vi "Create FPGA Data Node.vi"(6 "Path to Analog Node Template":string="IONode\\Analog Input Node x.vi", 7 "Values for Naming":T3={"Bus Number"=1, "Device Number"=1, "Channel Number"=1} {"Channel Number" min=1 step=1; "Device Number" min=1 step=1; "Bus Number" min=1 step=1}, 8 "error in":errorcluster, 10 "Device Information":T1={"Number of Channels"=1, "Device Alias"="", "Icon Text"={"Line 1 text"="Bus", "Line 2 text"="Dev", "Line 3 text"="Ch", "Line 4 text"=""}}, 11 "Path to IO Node":path=path "D:/Documents/Projects/SPIAPI/IOEngineCode") -> (0 "error out":errorcluster, 2 "IO Node Name":string, 3 "Path to new IO Node":path)   [LabVIEW 2014, in "SPI Engine Scripting.lvlib"]
doc: "Creates and saves an IO Node VI. It also modifies the values of its front panel controls based on the \"Values for Naming\" input."
uses:
  SPI Engine Scripting.lvlib
  State Machine/Controls/Values for Naming.ctl
  State Machine/Controls/Device Information.ctl
  <vilib>/LabVIEW Icon API/API_Text.ctl
  Icon Editor/Icon Editor.llb/Icon Colors.ctl
  <vilib>/LabVIEW Icon API/LabVIEW Icon API.lvlib
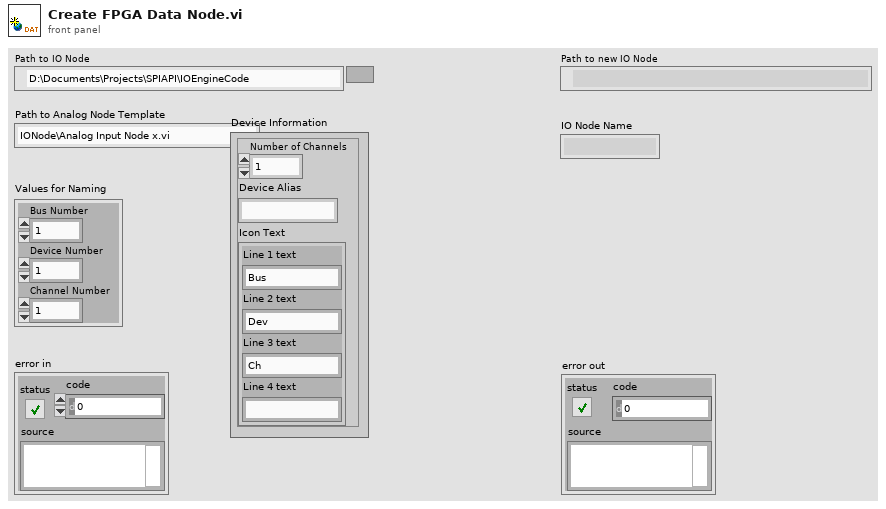
[diagram p1: front panel]
types:
  T1 = typedef "Device Information.ctl" = cluster{"Number of Channels":i32, "Device Alias":string, "Icon Text":T2}
  T2 = typedef "LabVIEW Icon API.lvlib/API_Text.ctl" = cluster{"Line 1 text":string, "Line 2 text":string, "Line 3 text":string, "Line 4 text":string}
  T3 = typedef "SPI Engine Scripting.lvlib/Values for Naming.ctl" = cluster{"Bus Number":i32, "Device Number":i32, "Channel Number":i32}
  T4 = typedef "Icon Colors.ctl" = cluster{"Text Color":u32, "Background Color":u32, "Border Color":u32}
  T5 = enum32{"invalid VI type", "Standard VI", "Control VI", "Global VI", "Polymorphic VI", "Configuration VI", "SubSystem", "Facade VI", "Method VI", "Statechart Diagram VI"}
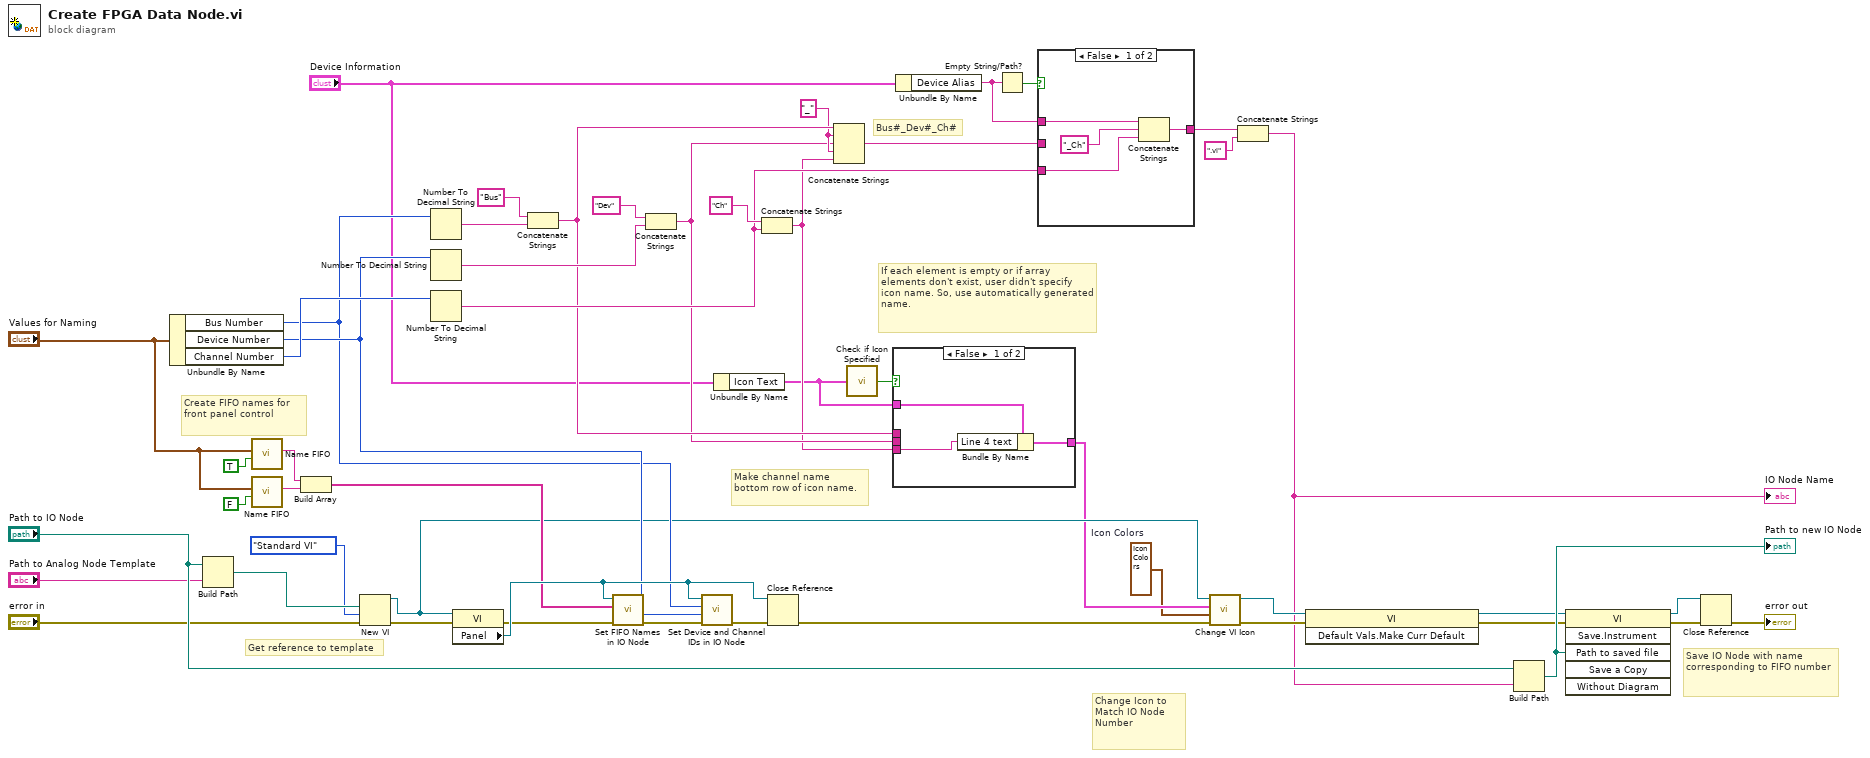
[diagram p0: block diagram]
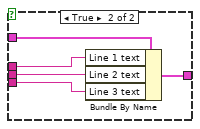
[diagram p3: hidden frame]
diagram:
  w22 = "_" ("string")
  w7 = T4 {"Text Color"=0, "Background Color"=16448250, "Border Color"=16746744}  # Icon Colors
  # "Make channel name bottom row of icon name."
  # "If each element is empty or if array elements don't exist, user didn't specify icon name. So, use automatically generated name."
  # "Bus#_Dev#_Ch#"
  # "Change Icon to Match IO Node Number"
  # "Get reference to template"
  # "Create FIFO names for front panel control"
  # "Save IO Node with name corresponding to FIFO number"
  n1 = Unbundle By Name("Values for Naming") -> ("Bus Number"=w31:i32, "Device Number"=w32:i32, "Channel Number"=w40:i32)
  n2 = Build Path(base path="Path to IO Node", name or relative path="Path to Analog Node Template") -> (appended path=w47:path)
  n3 = call "Name FIFO.vi"("TX?"=TRUE, "Values for Naming"="Values for Naming") -> ("FIFO Name"=w15:string)  [unwired: 9 in]
  n4 = call "Name FIFO.vi"("TX?"=FALSE, "Values for Naming"="Values for Naming") -> ("FIFO Name"=w14:string)  [unwired: 9 in]
  n5 = Build Array(w15, w14) -> (w13:string[])
  n6 = New VI(8:"error in", 9:T5."Standard VI" ("vi type (standard vi)"), 10:w47) -> (0:w50:errorcluster, 3:w9:refnum<vi>)  [unwired: 4 in]
  n7 = Number To Decimal String(number=w31) -> (decimal integer string=w34:string)  [unwired: 1 in]
  n8 = Number To Decimal String(number=w32) -> (decimal integer string=w33:string)  [unwired: 1 in]
  n9 = Number To Decimal String(number=w40) -> (decimal integer string=w28:string)  [unwired: 1 in]
  n10 = property class="VI"(reference=w9, error in=w50) -> (error out=w35:errorcluster, "Panel"=w36:refnum<vi>)  [unwired: 1 out]
  n11 = Concatenate Strings("Bus" ("string"), w34) -> (w23:string)
  n12 = call "Set FIFO Names in IO Node.vi"("error in (no error)"=w35, "Array"=w13, "Panel in"=w36) -> ("error out"=w30:errorcluster)  [unwired: 8 in]
  n13 = Concatenate Strings("Dev" ("string"), w33) -> (w21:string)
  n14 = call "Set Device and Channel IDs in IO Node.vi"("error in (no error)"=w30, "Device Number"=w32, "Bus Number"=w31, "Panel in"=w36) -> ("error out"=w29:errorcluster)  [unwired: 7 in]
  n15 = Unbundle By Name("Device Information") -> ("Icon Text"=w12:T2)
  n16 = Concatenate Strings("Ch" ("string"), w28) -> (w20:string)
  n17 = Close Reference(reference=w36, error in (no error)=w29) -> (error out=w6:errorcluster)
  n18 = Concatenate Strings(w23, w22, w21, w22, w20) -> (w19:string)
  n19 = call "Check if Icon Specified.vi"("Icon Text"=w12) -> ("No Icon Specified"=w25:bool)
  n20 = case shown="False" w25 {
    tunnel: w23 -> [_ w56]
    tunnel: w21 -> [_ w55]
    tunnel: w20 -> [w51 w54]
    tunnel: w12 -> [w52 w58]
    tunnel: [w53 w57] -> w8
    frame False {
      n21 = Bundle By Name(cluster=w52, "Line 4 text"=w51) -> (w53:T2)
    }
    frame True {
      n22 = Bundle By Name(cluster=w58, "Line 1 text"=w56, "Line 2 text"=w55, "Line 3 text"=w54) -> (w57:T2)
    }
  }
  n23 = Unbundle By Name("Device Information") -> ("Device Alias"=w11:string)
  n24 = Empty String/Path?(string/path=w11) -> (empty?=w24:bool)
  n25 = case shown="False" w24 {
    tunnel: [w62 w63] -> w2
    tunnel: w28 -> [w60 _]
    tunnel: w11 -> [w59 _]
    tunnel: w19 -> [_ w63]
    frame False {
      n26 = Concatenate Strings(w59, "_Ch" ("string"), w60) -> (w62:string)
    }
    frame True {
    }
  }
  n27 = call "Change VI Icon.vi"("Error In"=w6, "Icon Colors"=w7, "Icon Text"=w8, "Reference to VI In"=w9) -> ("Error Out"=w4:errorcluster, "Reference to VI Out"=w5:refnum<vi>)  [unwired: 6 in]
  n28 = Concatenate Strings(w2, ".vi" ("string")) -> (w1:string)
  "IO Node Name" <- w1
  n29 = invoke class="VI" method="Default Vals.Make Curr Default"(reference=w5, error in=w4) -> (reference out=w26:refnum<vi>, error out=w27:errorcluster)  [unwired: 1 in, 1 out]
  n30 = Build Path(base path="Path to IO Node", name or relative path=w1) -> (appended path=w46:path)
  "Path to new IO Node" <- w46
  n31 = invoke class="VI" method="Save.Instrument"(reference=w26, error in=w27, "Path to saved file"=w46) -> (reference out=w45:refnum<vi>, error out=w49:errorcluster)  [unwired: 3 in, 4 out]
  n32 = Close Reference(reference=w45, error in (no error)=w49) -> (error out=→"error out":errorcluster)
